vi "超标留样通讯.vi"(4 "value":u16, 6 "Slave ID":u8=2, 7 "STEP":T1(ring)=enum."read", 8 "Error in":errorcluster caption="Error in (no error)", 9 "values":u16[](array[numeric]), 10 "quantity":u16, 11 "starting address":u16 format="%04xH") -> (0 "error out":errorcluster, 2 "MB session in":refnum<class "MB_Master.lvclass">, 3 "Registers":u16[](array[numeric]))   [LabVIEW 2016, in "德润超标留样.lvlib"]
uses:
  <vilib>/Plasmionique/MB Master/MB_Master/MB_Master.lvclass
  <vilib>/Plasmionique/MB Master/MB_Master_Serial/MB_Master_Serial.lvclass
  D:/Program Files (x86)/National Instruments/LabVIEW 2016/vi.lib/Plasmionique/MB Master/MB_Master/MB_Master.lvclass
  <vilib>/Plasmionique/MB Master/MB_Master_TCP/MB_Master_TCP.lvclass
  <vilib>/Plasmionique/MB Master/MB Master.lvlib
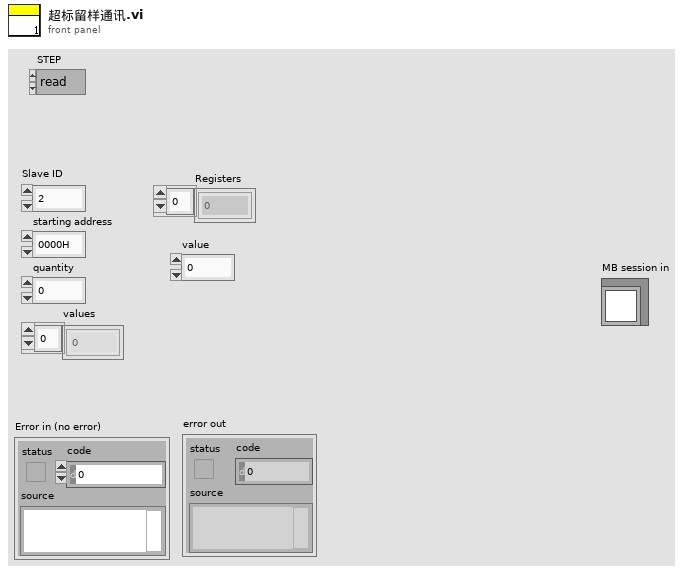
[diagram p1: front panel]
types:
  T1 = enum16{"open", "read", "write", "write single", "close"}
  T2 = cluster{"baud rate (bps)":u32, "stop bits":u16, "parity":u16, "flow control":u16, "timeout":u32, "retries":i32}
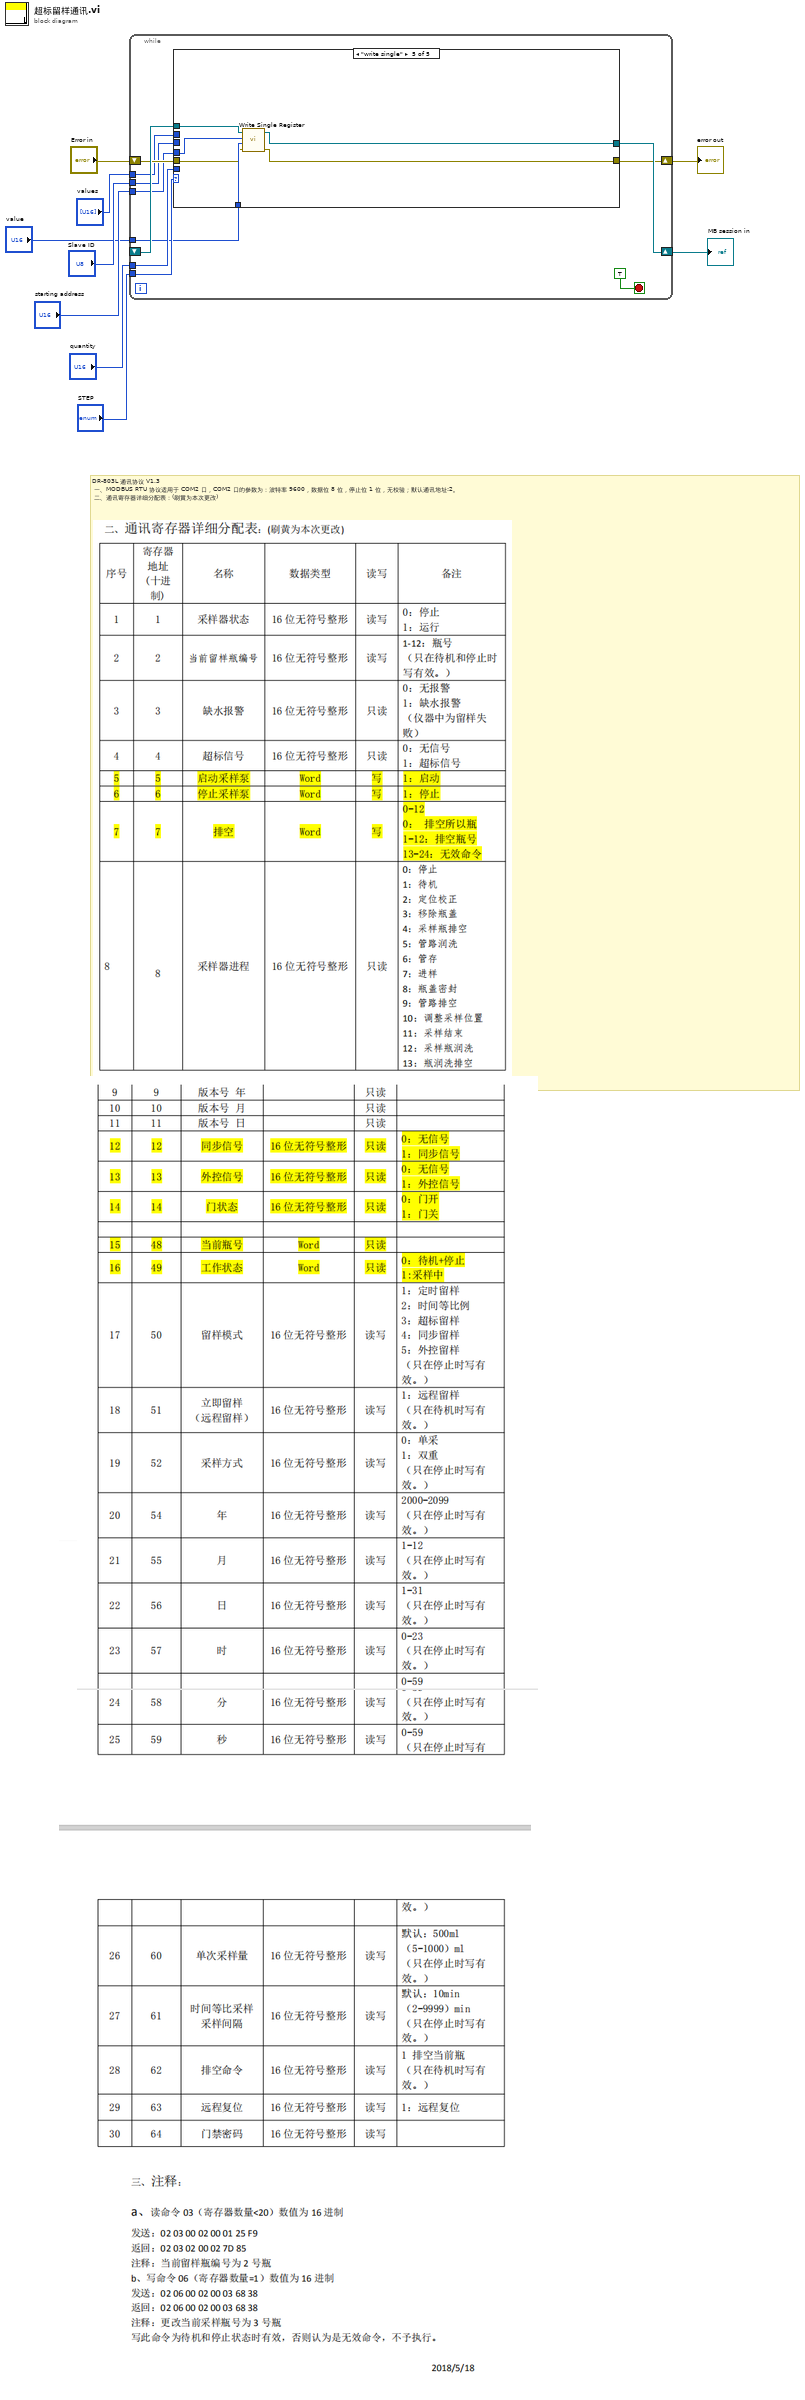
[diagram p0: block diagram]
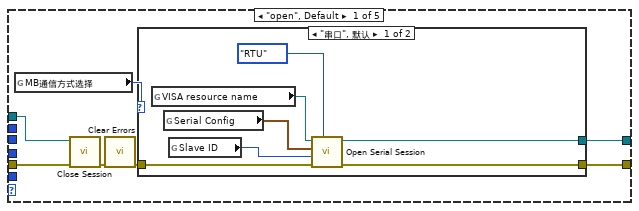
[diagram p2: hidden frame]
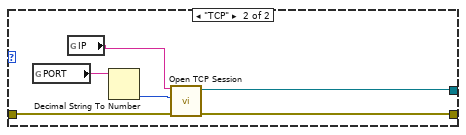
[diagram p3: hidden frame]
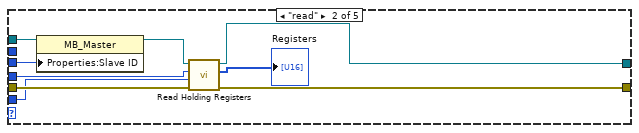
[diagram p4: hidden frame]
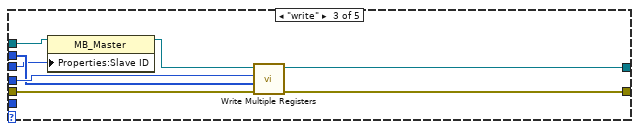
[diagram p5: hidden frame]
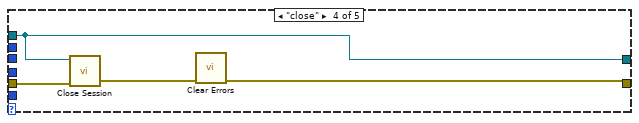
[diagram p6: hidden frame]
diagram:
  # "DR-803L 通讯协议 V1.3\n 一、MODBUS RTU 协议适用于 COM2 口，COM2 口的参数为：波特率 9600，数据位 8 位，停止位 1 位，无校验；默认通讯地址:2。\n 二、通讯寄存器详细分配表：(刷黄为本次更改)"
  n1 = while {
    shift-right: [w14] -> w2
    shift-left: _ -> [w20]
    shift-right: [w13] -> w8
    shift-left: "Error in" -> [w19]
    tunnel: "Slave ID" -> [w18]
    tunnel: "starting address" -> [w17]
    tunnel: "quantity" -> [w16]
    tunnel: "STEP" -> [w15]
    tunnel: "values" -> [w12]
    tunnel: "value" -> [w10]
    stop <- TRUE stop-if-true
    n2 = case shown="\"write single\"" w15 {
      tunnel: w20 -> [w25 w42 w52 w60 w67]
      tunnel: w19 -> [w24 w49 w57 w61 w62]
      tunnel: [w26 w48 w55 w60 w64] -> w14
      tunnel: [w27 w47 w56 w58 w63] -> w13
      tunnel: w18 -> [_ w45 w51 _ _]
      tunnel: w17 -> [_ w44 w54 _ w66]
      tunnel: w16 -> [_ w43 _ _ _]
      tunnel: w12 -> [_ _ w53 _ _]
      tunnel: w10 -> [_ _ _ _ w65]
      frame "open", Default {
        n3 = global read "串口参数断电保存全局变量.vi" "MB通信方式选择"() -> (w21:enum16{"串口", "TCP"})
        n4 = call-dynamic "Close Session.vi"("error in (no error)"=w24, "MB session in"=w25) -> ("error out"=w23:errorcluster)  [unwired: 9 in]
        n5 = call <vilib>:"Clear Errors.vi"("error in (no error)"=w23) -> ("error out"=w22:errorcluster)  [unwired: 5 in, 1 out]
        n6 = case shown="\"串口\", 默认" w21 {
          tunnel: [w33 w39] -> w27
          tunnel: [w28 w37] -> w26
          tunnel: w22 -> [w32 w38]
          frame "串口", Default {
            n7 = global read "串口参数断电保存全局变量.vi" "VISA resource name"() -> (w31:refnum<visa-resource-name>)
            n8 = global read "串口参数断电保存全局变量.vi" "Serial Config"() -> (w29:T2)
            n9 = global read "串口参数断电保存全局变量.vi" "Slave ID"() -> (w30:u8)
            n10 = call <vilib>:"Open Serial Session.vi"("Mode (RTU)"=enum16{"RTU", "ASCII"}."RTU", "Error in"=w32, "Slave ID"=w30, "Serial Config"=w29, "VISA Resource"=w31) -> ("Error out"=w33:errorcluster, "MB_Serial session"=w28:refnum<class "MB_Master_Serial.lvclass">)  [unwired: 5 in]
          }
          frame "TCP" {
            n11 = global read "串口参数断电保存全局变量.vi" "PORT"() -> (w35:string)
            n12 = global read "串口参数断电保存全局变量.vi" "IP"() -> (w36:string)
            n13 = Decimal String To Number(string=w35) -> (number=w40:i32)  [unwired: 2 in, 1 out]
            n14 = call <vilib>:"Open TCP Session.vi"("error in (no error)"=w38, "Port (502)"=w40, "IP Address"=w36) -> ("error out"=w39:errorcluster, "MB_TCP session"=w37:refnum<class "MB_Master_TCP.lvclass">)  [unwired: 7 in]
          }
        }
      }
      frame "read" {
        n15 = property class="MB_Master"(reference=w42, "Properties:Slave ID"=w45) -> (reference out=w41:refnum<class "MB_Master.lvclass">)  [unwired: 1 in, 1 out]
        n16 = call <vilib>:"Read Holding Registers.vi"("error in (no error)"=w49, "quantity"=w43, "starting address"=w44, "MB session in"=w41) -> ("error out"=w47:errorcluster, "Registers"=→"Registers":u16[], "MB session out"=w48:refnum<class "MB_Master.lvclass">)  [unwired: 5 in]
      }
      frame "write" {
        n17 = property class="MB_Master"(reference=w52, "Properties:Slave ID"=w51) -> (reference out=w50:refnum<class "MB_Master.lvclass">)  [unwired: 1 in, 1 out]
        n18 = call <vilib>:"Write Multiple Registers.vi"("error in (no error)"=w57, "values"=w53, "starting address"=w54, "MB session in"=w50) -> ("error out"=w56:errorcluster, "MB session out"=w55:refnum<class "MB_Master.lvclass">)  [unwired: 6 in]
      }
      frame "close" {
        n19 = call-dynamic "Close Session.vi"("error in (no error)"=w61, "MB session in"=w60) -> ("error out"=w59:errorcluster)  [unwired: 9 in]
        n20 = call <vilib>:"Clear Errors.vi"("error in (no error)"=w59) -> ("error out"=w58:errorcluster)  [unwired: 5 in, 1 out]
      }
      frame "write single" {
        n21 = call <vilib>:"Write Single Register.vi"("error in (no error)"=w62, "value"=w65, "address"=w66, "MB session in"=w67) -> ("error out"=w63:errorcluster, "MB session out"=w64:refnum<class "MB_Master.lvclass">)  [unwired: 6 in]
      }
    }
  }
  "error out" <- w8
  "MB session in" <- w2
